vi "Read property.vi"(11 "MsgSerializer.XMLProperty in":refnum<class "MsgSerializer.XML.lvclass">) -> (2 "format":T1=enum."property", 3 "MsgSerializer.XMLProperty out":refnum<class "MsgSerializer.XML.lvclass">)   [LabVIEW 2013, in "Caraya.lvlib" / "MsgSerializer.XML.lvclass"]
uses:
  MsgSerializer.XML.lvclass
  format -- enum.ctl
  MsgSerializer.XML.lvclass/MsgSerializer.XML.ctl
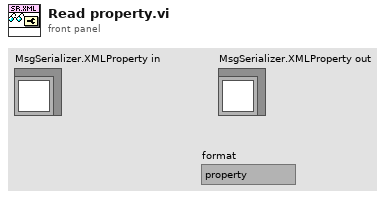
[diagram p1: front panel]
types:
  T1 = typedef "Caraya.lvlib/MsgSerializer.XML.lvclass/format -- enum.ctl" = enum16{"value", "tag", "property"}
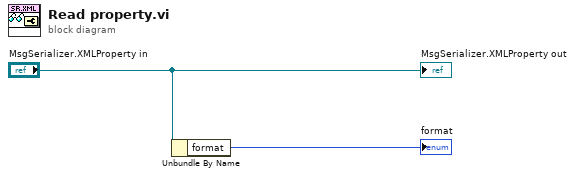
[diagram p0: block diagram]
diagram:
  n1 = Unbundle By Name("MsgSerializer.XMLProperty in") -> ("format"=→"format":T1)
  "MsgSerializer.XMLProperty out" <- "MsgSerializer.XMLProperty in"
